vi "AO Set.vi"(7 "Box ID":u8=1, 8 "error in (no error)":errorcluster, 9 "AO2 Voltage":dbl min=0.0 max=5.0, 10 "AO1 Voltage":dbl min=0.0 max=5.0, 11 "CAN in":refnum<class "XNET_BS120x.lvclass">) -> (0 "error out":errorcluster, 3 "CAN out":refnum<class "XNET_BS120x.lvclass">)   [LabVIEW 2021, in "BS120x Driver.lvlib" / "XNET_BS120x.lvclass"]
uses:
  XNET_BS120x.lvclass
  BS120x.lvclass
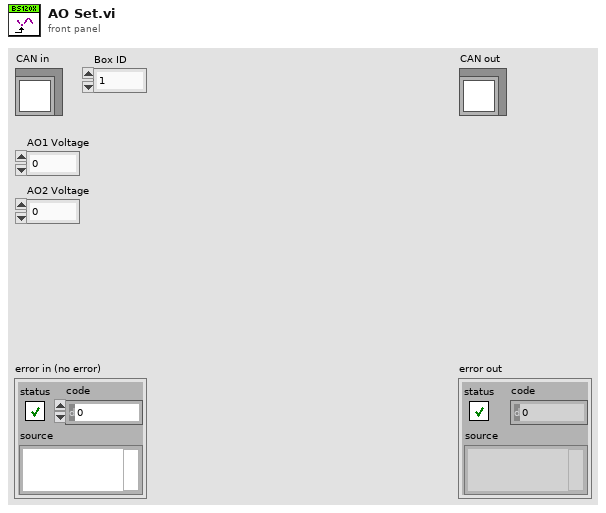
[diagram p1: front panel]
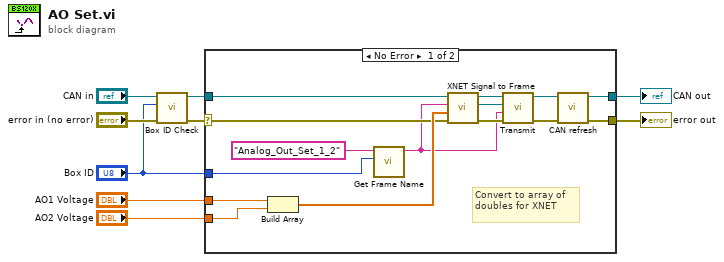
[diagram p0: block diagram]
diagram:
  n1 = call "Box ID Check.vi"("error in (no error)"="error in (no error)", "Box ID"="Box ID", "CAN in"="CAN in") -> ("error out"=w1:errorcluster, "CAN out"=w4:refnum<class "XNET_BS120x.lvclass">)  [unwired: 7 in]
  n2 = case shown="No Error" w1 {
    selector: w1 -> [w12 w26]
    tunnel: "AO1 Voltage" -> [w24 _]
    tunnel: "AO2 Voltage" -> [w23 _]
    tunnel: w4 -> [w20 w25]
    tunnel: [w16 w26] -> w6
    tunnel: [w14 w25] -> w5
    tunnel: "Box ID" -> [w13 _]
    frame No Error {
      # "Convert to array of doubles for XNET"
      n3 = Build Array(w24, w23) -> (w22:dbl[])
      n4 = call "Get Frame Name.vi"("Box ID"=w13, "Frame Name"="Analog_Out_Set_1_2" ("Frame")) -> ("Frame Name out"=w10:string)  [unwired: 9 in]
      n5 = call "XNET Signal to Frame.vi"("error in (no error)"=w12, "Data Array"=w22, "Frame"=w10, "CAN in"=w20) -> ("error out"=w21:errorcluster, "Data"=w19:refnum<class "XNET Data.lvclass">, "CAN out"=w18:refnum<class "XNET_BS120x.lvclass">)  [unwired: 5 in]
      n6 = call "Transmit.vi"("error in (no error)"=w21, "Frame"=w10, "Data in"=w19, "CAN in"=w18) -> ("error out"=w17:errorcluster, "CAN out"=w15:refnum<class "XNET_BS120x.lvclass">)  [unwired: 6 in]
      n7 = call "CAN refresh.vi"("error in (no error)"=w17, "CAN in"=w15) -> ("error out"=w16:errorcluster, "CAN out"=w14:refnum<class "XNET_BS120x.lvclass">)  [unwired: 8 in]
    }
    frame Error {
    }
  }
  "error out" <- w6
  "CAN out" <- w5
